vi "Period to RPM.vi"(1 "Period (sec)":dbl) -> (0 "Numeric Control":dbl)   [LabVIEW 2011]
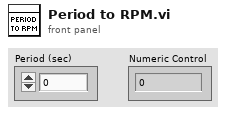
[diagram p1: front panel]
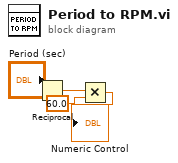
[diagram p0: block diagram]
diagram:
  n1 = Reciprocal(x="Period (sec)") -> (1/x=w1:dbl)
  n2 = Multiply(x=w1, y=60.0) -> (x*y=→"Numeric Control":dbl)
